vi "Measurement UI.vi"() -> ()   [LabVIEW 2021, in "audio_adc_frequencyResponseMeasurementUI.lvlib"]
uses:
  audio_adc_frequencyResponseMeasurementUI.lvlib
panel:
  in  "MeasGraphs":T1(tab)
  out "FrequencyResponseGraph":cluster{"X":dbl[], "Y":dbl[]}(graph) caption="AC"
  out "RMSLevelGraph":cluster{"X":dbl[], "Y":dbl[]}(graph) caption="AC"
  out "THDResponseGraph":cluster{"X":dbl[], "Y":dbl[]}(graph) caption="AC"
  out "THD+NResponseGraph":cluster{"X":dbl[], "Y":dbl[]}(graph) caption="AC"
  out "TimeDomainGraph":cluster{dbl, "dt":dbl, "Time domain":dbl[]}[](graph) caption="AC"
  in  "Bit clock edge sync":u32=1
  in  "Frame sync pulse width":u32=32
  in  "Frame length":u32=64
  in  "Data justification":u32 caption="Data Justification"
  in  "Endianness":u32
  in  "Channel 0 offset":u32=1
  in  "Bit depth":u32=24
  in  "Channel length":u32=32
  in  "Channel count per frame":u32=2
  in  "Frame sync edge for channel 0":u32=1
  out "Time domain plot sizes":i32[](array[numeric])
  out "THD+N response":dbl[](array[numeric])
  out "Frequency response":dbl[](array[numeric])
  out "Time domain":dbl[](array[numeric])
  out "dt":dbl
  out "RMS levels":dbl[](array[numeric])
  out "THD response":dbl[](array[numeric])
  out "Frequency steps":dbl[](array[numeric])
  in  "Configure Protocol Settings":bool
  in  "Analog source resource name":string(combo) caption="RESOURCE NAME"
  in  "Protocol capture resource name":string(combo) caption="RESOURCE NAME"
  in  "Data line":u16 caption="DATA LINE"
  in  "Channel":u32 caption="CHANNEL"
  in  "MeasSettingsOptions":i32(listbox)=-1
  in  "Settling time":dbl caption="SETTLING TIME" format="%#_6ps"
  in  "Settling cycles":i32 caption="SETTLING CYCLES"
  in  "Maximum harmonic":i32=5 caption="MAX HARMONIC"
  in  "DC Offset":dbl caption="DC OFFSET" format="%#_6pV"
  out "Protocol settings":string="Protocol settings"
  in  "Sample rate":dbl=44100.0 caption="SAMPLE RATE" format="%#.6pHz"
  in  "Frequency spacing":string(combo)="Logarithmic" caption="FREQUENCY SPACING"
  in  "Measurement duration":dbl=0.001 caption="MEASUREMENT DURATION" format="%#_6ps"
  in  "Measurement cycles":i32=10 caption="MEASUREMENT CYCLES"
  in  "Frequency steps":i32=20 caption="FREQUENCY STEPS"
  out "Analog source":string="Analog source "
  in  "Amplitude":dbl=-1.0 caption="AMPLITUDE" format="%#_6pdB"
  in  "Full scale range":dbl=2.825 caption="FULL SCALE RANGE" format="%.3pV"
  in  "Frequency stop":dbl=10000.0 caption="FREQUENCY STOP" format="%#_6pHz"
  in  "Frequency start":dbl=100.0 caption="FREQUENCY START" format="%#_6pHz"
  out "Measurement settings":string="Measurement settings"
  in  "MeasSettings":bool
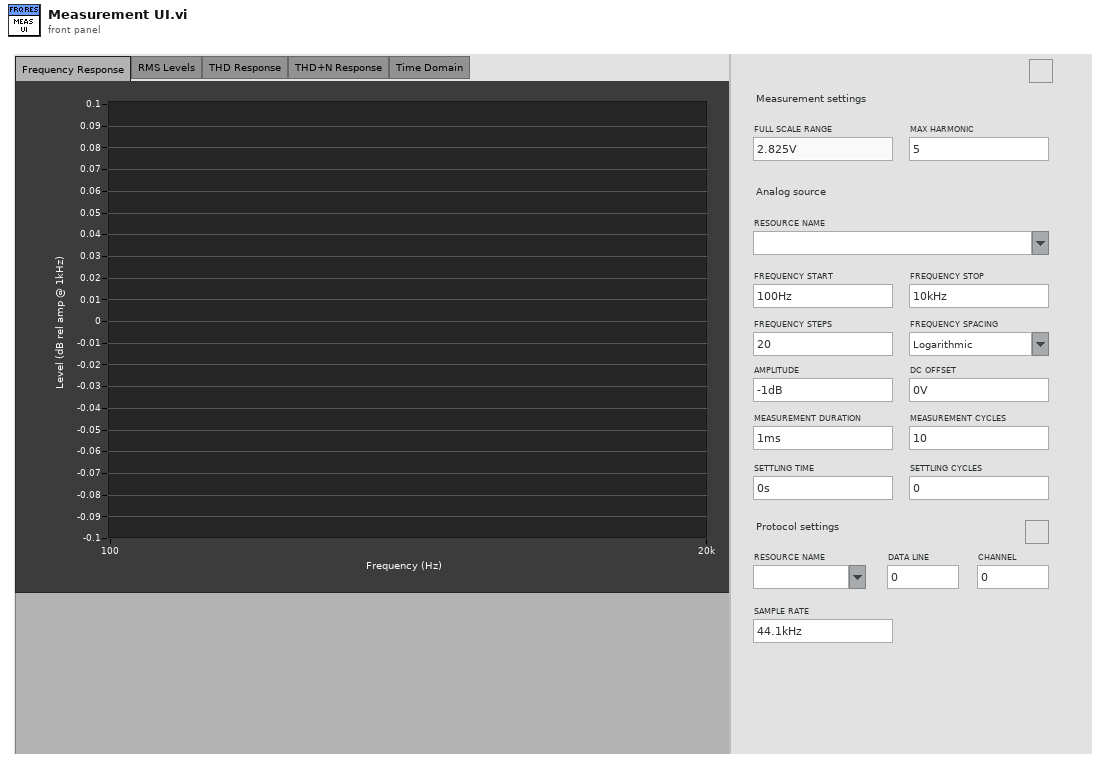
[diagram p1: front panel]
types:
  T1 = enum32{"Frequency Response", "RMS Levels", "THD Response", "THD+N Response", "Time Domain", "Hidden Controls"}
  T2 = enum16{"open", "replace", "create", "open or create", "replace or create", "replace or create with confirmation"}
  T3 = typedef "PDM Shared.lvlib/PCM Frame Sync Control.ctl" = cluster{"Frame Length":u16, "Frame Sync Pulse Width":u16, "Bit Clock Edge  Sync":T4}
  T4 = typedef "PDM Shared.lvlib/Digital Edge.ctl" = enum8{"Rising", "Falling"}
  T5 = typedef "PDM Shared.lvlib/PCM Data Format Configuration.ctl" = cluster{"Frame Sync Edge for Channel 0":T4, "Channel Count Per Frame":u8, "Channel Length":u16, "Bit Depth":u8, "Channel 0 Offset":u16, "Endianness":T6, "Data Justification":T7}
  T6 = typedef "PDM Shared.lvlib/PCM Bit Endianness.ctl" = enum16{"MSB First", "LSB First"}
  T7 = typedef "PDM Shared.lvlib/PCM Data Justification.ctl" = enum16{"Left Justified", "Right Justified"}
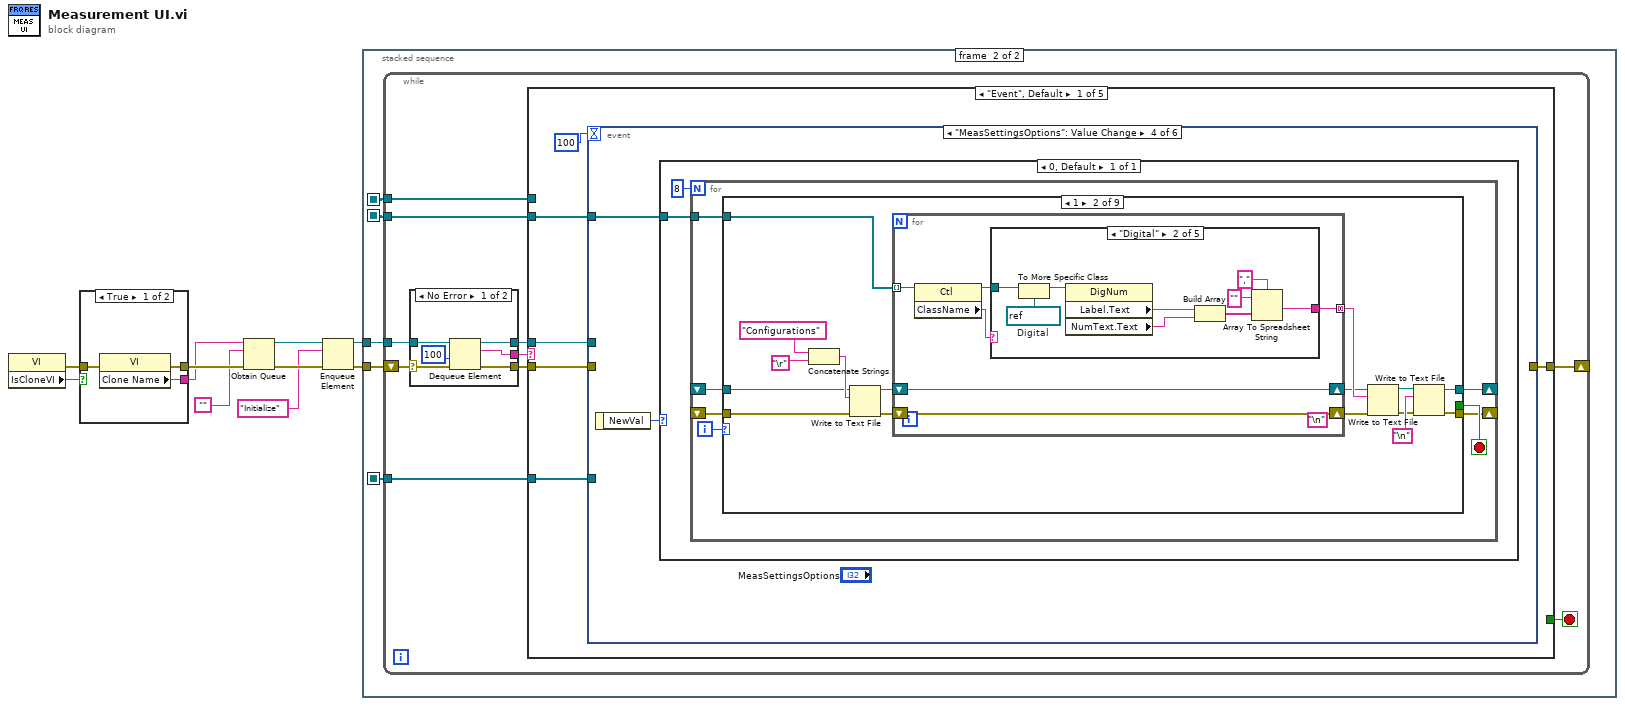
[diagram p0: block diagram]
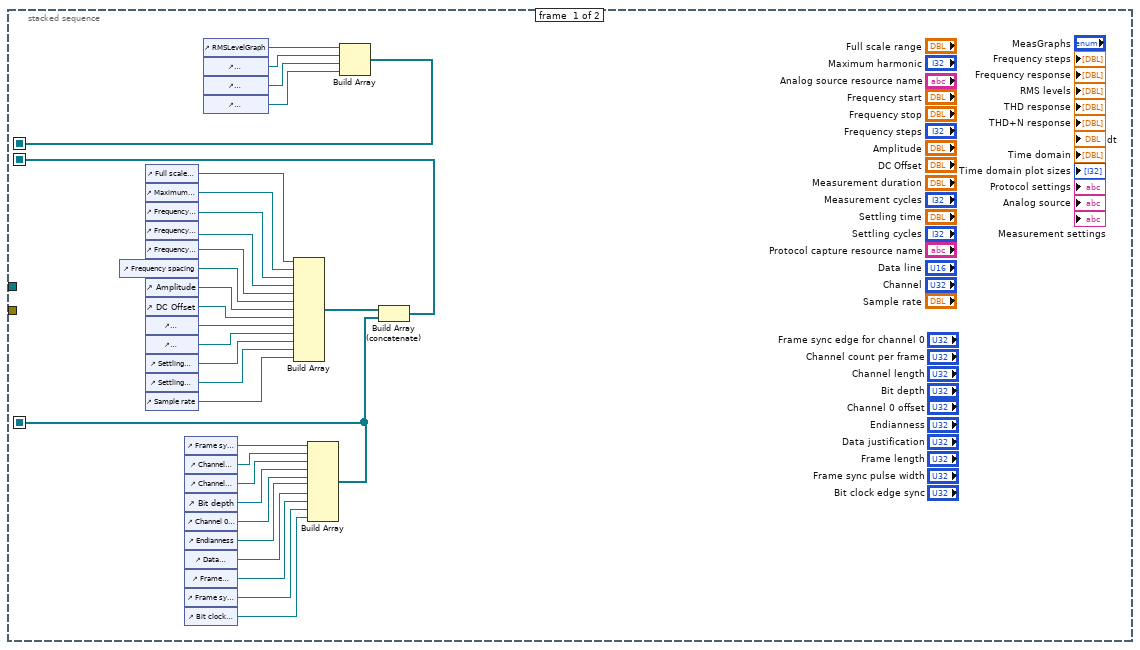
[diagram p2: hidden frame]
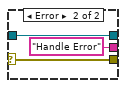
[diagram p3: hidden frame]
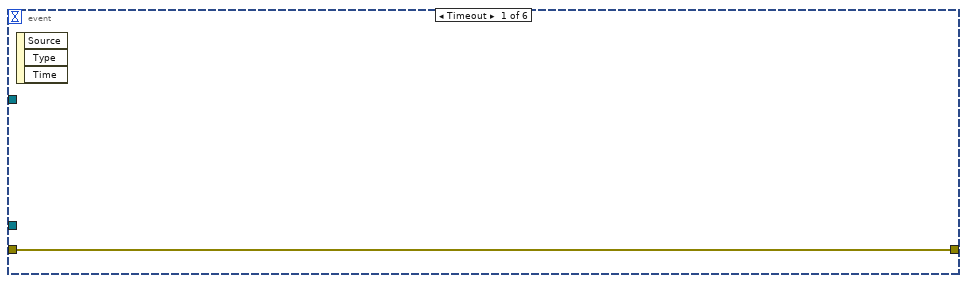
[diagram p4: hidden frame]
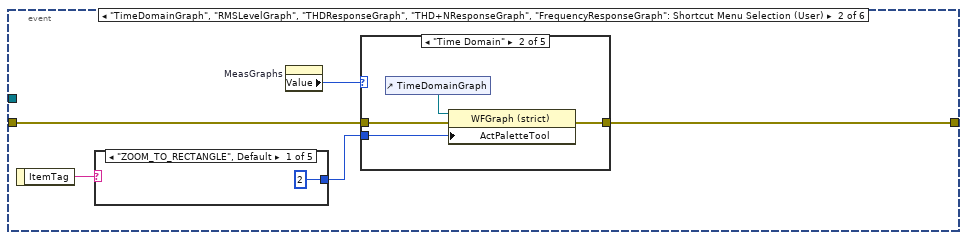
[diagram p5: hidden frame]
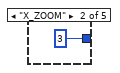
[diagram p6: hidden frame]
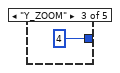
[diagram p7: hidden frame]
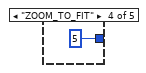
[diagram p8: hidden frame]
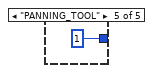
[diagram p9: hidden frame]
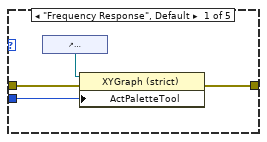
[diagram p10: hidden frame]
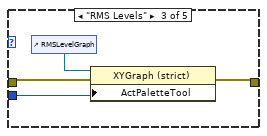
[diagram p11: hidden frame]
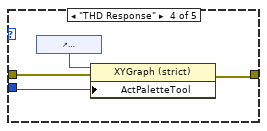
[diagram p12: hidden frame]
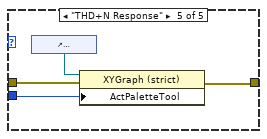
[diagram p13: hidden frame]
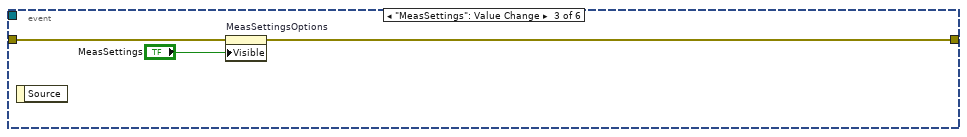
[diagram p14: hidden frame]
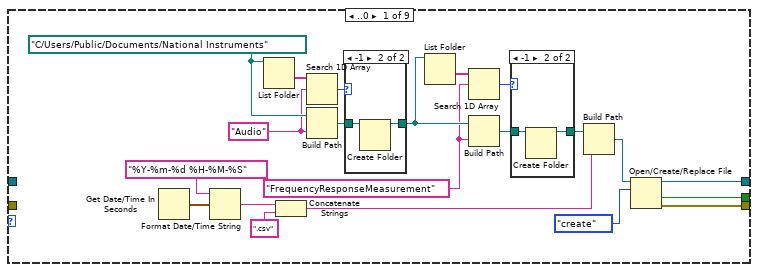
[diagram p15: hidden frame]
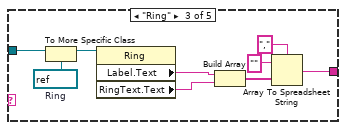
[diagram p19: hidden frame]
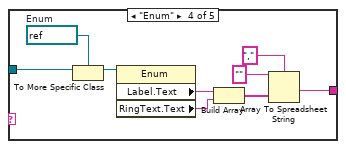
[diagram p20: hidden frame]
diagram:
  n1 = property class="VI"() -> (error out=w1:errorcluster, "IsCloneVI"=w2:bool)  [unwired: 2 in, 1 out]
  n2 = case shown="True" w2 {
    tunnel: [w13 w16] -> w10
    tunnel: [w12 w15] -> w9
    tunnel: w1 -> [w11 w14]
    frame True {
      n3 = property class="VI"(error in=w11) -> (error out=w13:errorcluster, "Clone Name"=w12:string)  [unwired: 1 in, 1 out]
    }
    frame False {
      n4 = property class="VI"(error in=w14) -> (error out=w16:errorcluster, "Name"=w15:string)  [unwired: 1 in, 1 out]
    }
  }
  n5 = Obtain Queue(name (unnamed)=w9, element data type="", error in (no error)=w10) -> (queue out=w6:refnum<queue>, error out=w8:errorcluster)  [unwired: 2 in, 1 out]
  n6 = Enqueue Element(queue=w6, element="Initialize", error in (no error)=w8) -> (queue out=w5:refnum<queue>, error out=w7:errorcluster)  [unwired: 1 in, 1 out]
  n7 = stacked-sequence {
    seq-local: [w18 _] -> [_ w48]
    seq-local: [w30 _] -> [_ w50]
    seq-local: [w17 _] -> [_ w49]
    tunnel: w7 -> [_ w52]
    tunnel: w5 -> [_ w51]
    frame #0 {
      n8 = control-ref of="Frequency spacing"() -> (w42:refnum<vi>)
      n9 = control-ref of="Full scale range"() -> (w47:refnum<vi>)
      n10 = control-ref of="Maximum harmonic"() -> (w46:refnum<vi>)
      n11 = control-ref of="Frequency start"() -> (w45:refnum<vi>)
      n12 = control-ref of="Frequency stop"() -> (w44:refnum<vi>)
      n13 = control-ref of="Frequency steps"() -> (w43:refnum<vi>)
      n14 = control-ref of="Amplitude"() -> (w36:refnum<vi>)
      n15 = control-ref of="DC Offset"() -> (w35:refnum<vi>)
      n16 = control-ref of="Measurement duration"() -> (w41:refnum<vi>)
      n17 = control-ref of="Measurement cycles"() -> (w40:refnum<vi>)
      n18 = control-ref of="Settling time"() -> (w39:refnum<vi>)
      n19 = control-ref of="Settling cycles"() -> (w38:refnum<vi>)
      n20 = control-ref of="Sample rate"() -> (w37:refnum<vi>)
      n21 = control-ref of="Frame sync edge for channel 0"() -> (w29:refnum<vi>)
      n22 = control-ref of="Channel count per frame"() -> (w28:refnum<vi>)
      n23 = control-ref of="Channel length"() -> (w27:refnum<vi>)
      n24 = control-ref of="Bit depth"() -> (w26:refnum<vi>)
      n25 = control-ref of="Channel 0 offset"() -> (w25:refnum<vi>)
      n26 = control-ref of="Endianness"() -> (w24:refnum<vi>)
      n27 = control-ref of="Data justification"() -> (w23:refnum<vi>)
      n28 = control-ref of="Frame length"() -> (w22:refnum<vi>)
      n29 = control-ref of="Frame sync pulse width"() -> (w21:refnum<vi>)
      n30 = control-ref of="Bit clock edge sync"() -> (w20:refnum<vi>)
      n31 = control-ref of="RMSLevelGraph"() -> (w34:refnum<vi>)
      n32 = control-ref of="THDResponseGraph"() -> (w33:refnum<vi>)
      n33 = control-ref of="THD+NResponseGraph"() -> (w32:refnum<vi>)
      n34 = control-ref of="FrequencyResponseGraph"() -> (w31:refnum<vi>)
      n35 = Build Array(w47, w46, w45, w44, w43, w42, w36, w35, w41, w40, w39, w38, w37) -> (w19:refnum<vi>[])
      n36 = Build Array(w29, w28, w27, w26, w25, w24, w23, w22, w21, w20) -> (w17:refnum<vi>[])
      n37 = Build Array(w34, w33, w32, w31) -> (w30:refnum<vi>[])
      n38 = Build Array (concatenate)(w19, w17) -> (w18:refnum<vi>[])
    }
    frame #1 {
      n39 = while {
        shift-right: [w57] -> _
        shift-left: w52 -> [w62]
        tunnel: w51 -> [w60]
        tunnel: w50 -> [w55]
        tunnel: w49 -> [w54]
        tunnel: w48 -> [w53]
        stop <- w56 stop-if-true
        n40 = case shown="No Error" w62 {
          selector: w62 -> [w68 w71]
          tunnel: [w67 w71] -> w61
          tunnel: w60 -> [w66 w70]
          tunnel: [w65 w70] -> w59
          tunnel: [w64 "Handle Error"] -> w58
          frame No Error {
            n41 = Dequeue Element(queue=w66, timeout in ms (-1)=100, error in (no error)=w68) -> (queue out=w65:refnum<queue>, element=w64:string, error out=w67:errorcluster)  [unwired: 1 out]
          }
          frame Error {
          }
        }
        n42 = case shown="\"Event\", Default" w58 {
          tunnel: w61 -> [w76 w394 w431 w458 w459]
          tunnel: w59 -> [w74 _ _ w456 _]
          tunnel: [w77 w394 w431 w453 w459] -> w57
          tunnel: [_ _ _ TRUE _] -> w56
          tunnel: w55 -> [_ _ w405 _ _]
          tunnel: w54 -> [w73 _ _ _ _]
          tunnel: w53 -> [w72 _ _ _ _]
          frame "Event", Default {
            n43 = event shown="[3] \"MeasSettingsOptions\": Value Change" {
              selector: _ -> [_ _ _ _ _ _]
              dyn-events: _ -> [_ _ _ _ _ _]
              timeout: 100 -> [_ _ _ _ _ _]
              tunnel: [w78 w79 w109 _ w381 w384] -> w77
              tunnel: w76 -> [w78 w81 w111 _ w381 w385]
              tunnel: w74 -> [_ _ _ _ _ w383]
              tunnel: w73 -> [_ _ _ _ w378 _]
              tunnel: w72 -> [_ _ _ w112 _ _]
              event Timeout {
                n44 = event-data() -> ()  [unwired: 1 in, 3 out]
              }
              event "TimeDomainGraph", "RMSLevelGraph", "THDResponseGraph", "THD+NResponseGraph", "FrequencyResponseGraph": Shortcut Menu Selection (User) {
                n45 = event-data() -> ("ItemTag"=w82:string)  [unwired: 1 in]
                n46 = case shown="\"ZOOM_TO_RECTANGLE\", Default" w82 {
                  tunnel: [2 3 4 5 1] -> w80
                  frame "ZOOM_TO_RECTANGLE", Default {
                  }
                  frame "X_ZOOM" {
                  }
                  frame "Y_ZOOM" {
                  }
                  frame "ZOOM_TO_FIT" {
                  }
                  frame "PANNING_TOOL" {
                  }
                }
                n47 = property on="MeasGraphs" class="TabCtl (strict)"() -> ("Value"=w83:T1)  [unwired: 2 in, 2 out]
                n48 = case shown="\"Time Domain\"" w83 {
                  tunnel: w81 -> [w92 w95 w99 w104 w108]
                  tunnel: w80 -> [w89 w94 w98 w101 w107]
                  tunnel: [w91 w93 w97 w103 w106] -> w79
                  frame "Frequency Response", Default {
                    n49 = control-ref of="FrequencyResponseGraph"() -> (w90:refnum<vi>)
                    n50 = property class="XYGraph (strict)"(reference=w90, error in=w92, "ActPaletteTool"=w89) -> (error out=w91:errorcluster)  [unwired: 1 out]
                  }
                  frame "Time Domain" {
                    n51 = control-ref of="TimeDomainGraph"() -> (w96:refnum<vi>)
                    n52 = property class="WFGraph (strict)"(reference=w96, error in=w95, "ActPaletteTool"=w94) -> (error out=w93:errorcluster)  [unwired: 1 out]
                  }
                  frame "RMS Levels" {
                    n53 = control-ref of="RMSLevelGraph"() -> (w100:refnum<vi>)
                    n54 = property class="XYGraph (strict)"(reference=w100, error in=w99, "ActPaletteTool"=w98) -> (error out=w97:errorcluster)  [unwired: 1 out]
                  }
                  frame "THD Response" {
                    n55 = control-ref of="THDResponseGraph"() -> (w102:refnum<vi>)
                    n56 = property class="XYGraph (strict)"(reference=w102, error in=w104, "ActPaletteTool"=w101) -> (error out=w103:errorcluster)  [unwired: 1 out]
                  }
                  frame "THD+N Response" {
                    n57 = control-ref of="THD+NResponseGraph"() -> (w105:refnum<vi>)
                    n58 = property class="XYGraph (strict)"(reference=w105, error in=w108, "ActPaletteTool"=w107) -> (error out=w106:errorcluster)  [unwired: 1 out]
                  }
                }
              }
              event "MeasSettings": Value Change {
                n59 = event-data() -> ()  [unwired: 1 in, 1 out]
                n60 = property on="MeasSettingsOptions" class="LstBox (strict)"(error in=w111, "Visible"="MeasSettings") -> (error out=w109:errorcluster)  [unwired: 1 in, 1 out]
              }
              event "MeasSettingsOptions": Value Change {
                n61 = event-data() -> ("NewVal"=w113:i32)  [unwired: 1 in]
                n62 = case shown="0, Default" w113 {
                  tunnel: w112 -> [w114]
                  frame 0, Default {
                    n63 = for {
                      N: 8 -> [_]
                      shift-right: [w120] -> _
                      shift-left: _ -> [w119]
                      shift-right: [w118] -> _
                      shift-left: _ -> [w117]
                      tunnel: w114 -> [w116]
                      i -> [w122]
                      stop <- w121 stop-if-true
                      n64 = case shown="1" w122 {
                        tunnel: [w136 _ _ _ _ _ _ _ _] -> w121
                        tunnel: [w142 w151 w215 w246 w278 w310 w340 refnum<file> refnum ("refnum out") w377] -> w120
                        tunnel: w119 -> [_ w162 w235 w267 w299 w331 w348 w375 w377]
                        tunnel: [w135 w152 w213 w244 w276 w308 w339 w373 w376] -> w118
                        tunnel: w117 -> [_ w160 w234 w266 w298 w330 w349 w372 w376]
                        tunnel: w116 -> [_ w150 _ _ _ _ _ _ _]
                        frame ..0 {
                          w131 = "FrequencyResponseMeasurement" ("prompt")
                          w138 = "Audio" ("prompt")
                          w141 = path "C:/Users/Public/Documents/National Instruments" ("base path")
                          n65 = Get Date/Time In Seconds() -> (seconds since 1Jan1904=w128:timestamp)
                          n66 = Format Date/Time String(time format string (%c)="%Y-%m-%d %H-%M-%S", seconds (now)=w128) -> (date/time string=w127:string)  [unwired: 1 in]
                          n67 = List Folder(path=w141) -> (folder names=w139:string[])  [unwired: 3 in, 3 out]
                          n68 = Concatenate Strings(w127, ".csv" ("string")) -> (w124:string)
                          n69 = Search 1D Array(1D array=w139, element=w138) -> (index of element=w137:i32)  [unwired: 1 in]
                          n70 = Build Path(base path=w141, name or relative path=w138) -> (appended path=w140:path)
                          n71 = case shown="-1" w137 {
                            tunnel: w140 -> [w147 w149]
                            tunnel: [w147 w148] -> w132
                            frame Default {
                            }
                            frame -1 {
                              n72 = Create Folder(path (use dialog)=w149) -> (created path=w148:path)  [unwired: 2 in, 2 out]
                            }
                          }
                          n73 = List Folder(path=w132) -> (folder names=w134:string[])  [unwired: 3 in, 3 out]
                          n74 = Search 1D Array(1D array=w134, element=w131) -> (index of element=w133:i32)  [unwired: 1 in]
                          n75 = Build Path(base path=w132, name or relative path=w131) -> (appended path=w130:path)
                          n76 = case shown="-1" w133 {
                            tunnel: w130 -> [w144 w146]
                            tunnel: [w144 w145] -> w125
                            frame Default {
                            }
                            frame -1 {
                              n77 = Create Folder(path (use dialog)=w146) -> (created path=w145:path)  [unwired: 2 in, 2 out]
                            }
                          }
                          n78 = Build Path(base path=w125, name or relative path=w124) -> (appended path=w123:path)
                          n79 = Open/Create/Replace File(file path (use dialog)=w123, operation (0:open)=T2."create") -> (refnum out=w142:refnum<file>, cancelled=w136:bool, error out=w135:errorcluster)  [unwired: 4 in]
                        }
                        frame 1 {
                          (unwired) "\n"
                          n80 = Concatenate Strings("Configurations" ("format string"), "\r") -> (w163:string)
                          n81 = Write to Text File(file (use dialog)=w162, text=w163, error in=w160) -> (refnum out=w159:refnum<file>, error out=w161:errorcluster)  [unwired: 1 in, 1 out]
                          n82 = for {
                            shift-right: [w171] -> w157
                            shift-left: w159 -> [w171]
                            shift-right: [w170] -> w156
                            shift-left: w161 -> [w170]
                            tunnel: [w169] -> w158 mode=concatenating
                            tunnel: w150 -> [w166] mode=indexing
                            n83 = property class="Ctl"(reference=w166) -> (reference out=w168:refnum<vi>, "ClassName"=w167:string)  [unwired: 1 in, 1 out]
                            n84 = case shown="\"Digital\"" w167 {
                              tunnel: [_ w175 w185 w194 w203] -> w169
                              tunnel: w168 -> [_ w173 w183 w198 w207]
                              frame Default {
                              }
                              frame "Digital" {
                                w172 = refnum<vi> refnum  # Digital
                                n85 = To More Specific Class(target class=w172, reference=w173) -> (specific class reference=w174:refnum<vi>)  [unwired: 1 in, 1 out]
                                n86 = property class="DigNum"(reference=w174) -> ("Label.Text"=w180:string, "NumText.Text"=w179:string)  [unwired: 1 in, 2 out]
                                n87 = Build Array(w180, w179) -> (w176:string[])
                                n88 = Array To Spreadsheet String(delimiter (Tab)=",", array=w176, 3:"" ("format string")) -> (spreadsheet string=w175:string)
                              }
                              frame "Ring" {
                                w182 = refnum<vi> refnum  # Ring
                                n89 = To More Specific Class(target class=w182, reference=w183) -> (specific class reference=w184:refnum<vi>)  [unwired: 1 in, 1 out]
                                n90 = property class="Ring"(reference=w184) -> ("Label.Text"=w181:string, "RingText.Text"=w189:string)  [unwired: 1 in, 2 out]
                                n91 = Build Array(w181, w189) -> (w186:string[])
                                n92 = Array To Spreadsheet String(delimiter (Tab)=",", array=w186, 3:"" ("format string")) -> (spreadsheet string=w185:string)
                              }
                              frame "Enum" {
                                w197 = refnum<vi> refnum  # Enum
                                n93 = To More Specific Class(target class=w197, reference=w198) -> (specific class reference=w193:refnum<vi>)  [unwired: 1 in, 1 out]
                                n94 = property class="Enum"(reference=w193) -> ("Label.Text"=w192:string, "RingText.Text"=w191:string)  [unwired: 1 in, 2 out]
                                n95 = Build Array(w192, w191) -> (w190:string[])
                                n96 = Array To Spreadsheet String(delimiter (Tab)=",", array=w190, 3:"" ("format string")) -> (spreadsheet string=w194:string)
                              }
                              frame "ComboBox" {
                                w206 = refnum<vi> refnum  # ComboBox
                                n97 = To More Specific Class(target class=w206, reference=w207) -> (specific class reference=w202:refnum<vi>)  [unwired: 1 in, 1 out]
                                n98 = property class="CmbBox"(reference=w202) -> ("Label.Text"=w201:string, "Value"=w200:string)  [unwired: 1 in, 2 out]
                                n99 = Build Array(w201, w200) -> (w199:string[])
                                n100 = Array To Spreadsheet String(delimiter (Tab)=",", array=w199, 3:"" ("format string")) -> (spreadsheet string=w203:string)
                              }
                            }
                          }
                          n101 = Write to Text File(file (use dialog)=w157, text=w158, error in=w156) -> (refnum out=w154:refnum<file>, error out=w153:errorcluster)  [unwired: 1 in, 1 out]
                          n102 = Write to Text File(file (use dialog)=w154, text="\n", error in=w153) -> (refnum out=w151:refnum<file>, error out=w152:errorcluster)  [unwired: 1 in, 1 out]
                        }
                        frame 2 {
                          w208 = "\r"
                          n103 = property on="FrequencyResponseGraph" class="XYGraph (strict)"() -> ("Value"=w210:cluster{"X":dbl[], "Y":dbl[]})  [unwired: 2 in, 2 out]
                          n104 = Concatenate Strings("Results" ("string"), w208, "Frequency Response" ("string"), w208) -> (w232:string)
                          n105 = Write to Text File(file (use dialog)=w235, text=w232, error in=w234) -> (refnum out=w228:refnum<file>, error out=w227:errorcluster)  [unwired: 1 in, 1 out]
                          n106 = Build Array("Frequency (Hz)", "Level (dB rel amp @ 1kHz)") -> (w231:string[])
                          n107 = Unbundle By Name(w210) -> ("X"=w219:dbl[], "Y"=w220:dbl[])
                          n108 = Array To Spreadsheet String(delimiter (Tab)=",", array=w231, 3:"" ("format string")) -> (spreadsheet string=w226:string)
                          n109 = for {
                            tunnel: w219 -> [w240] mode=indexing
                            tunnel: w220 -> [w236] mode=indexing
                            tunnel: [w237] -> w221 mode=indexing
                            n110 = Format Into String(w240) -> (resulting string=w238:string)  [unwired: 3 in, 1 out]
                            n111 = Format Into String(w236) -> (resulting string=w239:string)  [unwired: 3 in, 1 out]
                            n112 = Build Array(w238, w239) -> (w237:string[])
                          }
                          n113 = Write to Text File(file (use dialog)=w228, text=w226, error in=w227) -> (refnum out=w225:refnum<file>, error out=w224:errorcluster)  [unwired: 1 in, 1 out]
                          n114 = Array To Spreadsheet String(delimiter (Tab)=",", array=w221, 3:"" ("format string")) -> (spreadsheet string=w218:string)
                          n115 = Write to Text File(file (use dialog)=w225, text=w218, error in=w224) -> (refnum out=w217:refnum<file>, error out=w216:errorcluster)  [unwired: 1 in, 1 out]
                          n116 = Write to Text File(file (use dialog)=w217, text="\n", error in=w216) -> (refnum out=w215:refnum<file>, error out=w213:errorcluster)  [unwired: 1 in, 1 out]
                        }
                        frame 3 {
                          n117 = property on="RMSLevelGraph" class="XYGraph (strict)"() -> ("Value"=w241:cluster{"X":dbl[], "Y":dbl[]})  [unwired: 2 in, 2 out]
                          n118 = Concatenate Strings("RMS Level" ("string"), "\r") -> (w264:string)
                          n119 = Build Array("Frequency (Hz)", "Level (Vrms)") -> (w263:string[])
                          n120 = Write to Text File(file (use dialog)=w267, text=w264, error in=w266) -> (refnum out=w260:refnum<file>, error out=w259:errorcluster)  [unwired: 1 in, 1 out]
                          n121 = Array To Spreadsheet String(delimiter (Tab)=",", array=w263, 3:"" ("format string")) -> (spreadsheet string=w258:string)
                          n122 = Unbundle By Name(w241) -> ("X"=w251:dbl[], "Y"=w252:dbl[])
                          n123 = Write to Text File(file (use dialog)=w260, text=w258, error in=w259) -> (refnum out=w257:refnum<file>, error out=w256:errorcluster)  [unwired: 1 in, 1 out]
                          n124 = for {
                            tunnel: w251 -> [w272] mode=indexing
                            tunnel: w252 -> [w268] mode=indexing
                            tunnel: [w269] -> w253 mode=indexing
                            n125 = Format Into String(w272) -> (resulting string=w270:string)  [unwired: 3 in, 1 out]
                            n126 = Format Into String(w268) -> (resulting string=w271:string)  [unwired: 3 in, 1 out]
                            n127 = Build Array(w270, w271) -> (w269:string[])
                          }
                          n128 = Array To Spreadsheet String(delimiter (Tab)=",", array=w253, 3:"" ("format string")) -> (spreadsheet string=w250:string)
                          n129 = Write to Text File(file (use dialog)=w257, text=w250, error in=w256) -> (refnum out=w248:refnum<file>, error out=w247:errorcluster)  [unwired: 1 in, 1 out]
                          n130 = Write to Text File(file (use dialog)=w248, text="\n", error in=w247) -> (refnum out=w246:refnum<file>, error out=w244:errorcluster)  [unwired: 1 in, 1 out]
                        }
                        frame 4 {
                          n131 = Concatenate Strings("THD Response" ("string"), "\r") -> (w296:string)
                          n132 = property on="THDResponseGraph" class="XYGraph (strict)"() -> ("Value"=w273:cluster{"X":dbl[], "Y":dbl[]})  [unwired: 2 in, 2 out]
                          n133 = Build Array("Frequency (Hz)", "THD (dB)") -> (w295:string[])
                          n134 = Write to Text File(file (use dialog)=w299, text=w296, error in=w298) -> (refnum out=w292:refnum<file>, error out=w291:errorcluster)  [unwired: 1 in, 1 out]
                          n135 = Array To Spreadsheet String(delimiter (Tab)=",", array=w295, 3:"" ("format string")) -> (spreadsheet string=w290:string)
                          n136 = Unbundle By Name(w273) -> ("X"=w283:dbl[], "Y"=w284:dbl[])
                          n137 = Write to Text File(file (use dialog)=w292, text=w290, error in=w291) -> (refnum out=w289:refnum<file>, error out=w288:errorcluster)  [unwired: 1 in, 1 out]
                          n138 = for {
                            tunnel: w283 -> [w304] mode=indexing
                            tunnel: w284 -> [w300] mode=indexing
                            tunnel: [w301] -> w285 mode=indexing
                            n139 = Format Into String(w304) -> (resulting string=w302:string)  [unwired: 3 in, 1 out]
                            n140 = Format Into String(w300) -> (resulting string=w303:string)  [unwired: 3 in, 1 out]
                            n141 = Build Array(w302, w303) -> (w301:string[])
                          }
                          n142 = Array To Spreadsheet String(delimiter (Tab)=",", array=w285, 3:"" ("format string")) -> (spreadsheet string=w282:string)
                          n143 = Write to Text File(file (use dialog)=w289, text=w282, error in=w288) -> (refnum out=w280:refnum<file>, error out=w279:errorcluster)  [unwired: 1 in, 1 out]
                          n144 = Write to Text File(file (use dialog)=w280, text="\n", error in=w279) -> (refnum out=w278:refnum<file>, error out=w276:errorcluster)  [unwired: 1 in, 1 out]
                        }
                        frame 5 {
                          n145 = property on="THD+NResponseGraph" class="XYGraph (strict)"() -> ("Value"=w305:cluster{"X":dbl[], "Y":dbl[]})  [unwired: 2 in, 2 out]
                          n146 = Concatenate Strings("THD+N Response" ("string"), "\r") -> (w328:string)
                          n147 = Build Array("Frequency (Hz)", "THD+N (dB)") -> (w327:string[])
                          n148 = Write to Text File(file (use dialog)=w331, text=w328, error in=w330) -> (refnum out=w324:refnum<file>, error out=w323:errorcluster)  [unwired: 1 in, 1 out]
                          n149 = Array To Spreadsheet String(delimiter (Tab)=",", array=w327, 3:"" ("format string")) -> (spreadsheet string=w322:string)
                          n150 = Unbundle By Name(w305) -> ("X"=w315:dbl[], "Y"=w316:dbl[])
                          n151 = Write to Text File(file (use dialog)=w324, text=w322, error in=w323) -> (refnum out=w321:refnum<file>, error out=w320:errorcluster)  [unwired: 1 in, 1 out]
                          n152 = for {
                            tunnel: w315 -> [w336] mode=indexing
                            tunnel: w316 -> [w332] mode=indexing
                            tunnel: [w333] -> w317 mode=indexing
                            n153 = Format Into String(w336) -> (resulting string=w334:string)  [unwired: 3 in, 1 out]
                            n154 = Format Into String(w332) -> (resulting string=w335:string)  [unwired: 3 in, 1 out]
                            n155 = Build Array(w334, w335) -> (w333:string[])
                          }
                          n156 = Array To Spreadsheet String(delimiter (Tab)=",", array=w317, 3:"" ("format string")) -> (spreadsheet string=w314:string)
                          n157 = Write to Text File(file (use dialog)=w321, text=w314, error in=w320) -> (refnum out=w312:refnum<file>, error out=w311:errorcluster)  [unwired: 1 in, 1 out]
                          n158 = Write to Text File(file (use dialog)=w312, text="\n", error in=w311) -> (refnum out=w310:refnum<file>, error out=w308:errorcluster)  [unwired: 1 in, 1 out]
                        }
                        frame 6 {
                          n159 = Concatenate Strings("Time Domain" ("string"), "\r") -> (w361:string)
                          n160 = Write to Text File(file (use dialog)=w348, text=w361, error in=w349) -> (refnum out=w358:refnum<file>, error out=w357:errorcluster)  [unwired: 1 in, 1 out]
                          n161 = Build Array("Time (s)", "Amplitude (V)") -> (w360:string[])
                          n162 = property on="dt" class="DigNum (strict)"() -> ("Value"=w337:dbl)  [unwired: 2 in, 2 out]
                          n163 = property on="Time domain" class="Arr (strict)"() -> ("Value"=w338:dbl[])  [unwired: 2 in, 2 out]
                          n164 = Array To Spreadsheet String(delimiter (Tab)=",", array=w360, 3:"" ("format string")) -> (spreadsheet string=w356:string)
                          n165 = Write to Text File(file (use dialog)=w358, text=w356, error in=w357) -> (refnum out=w355:refnum<file>, error out=w354:errorcluster)  [unwired: 1 in, 1 out]
                          n166 = for {
                            tunnel: [w367] -> w351 mode=indexing
                            tunnel: w338 -> [w366] mode=indexing
                            tunnel: w337 -> [w364]
                            i -> [w365]
                            n167 = Multiply(x=w364, y=w365) -> (x*y=w363:dbl)
                            n168 = Format Into String(w363) -> (resulting string=w368:string)  [unwired: 3 in, 1 out]
                            n169 = Format Into String(w366) -> (resulting string=w369:string)  [unwired: 3 in, 1 out]
                            n170 = Build Array(w368, w369) -> (w367:string[])
                          }
                          n171 = Array To Spreadsheet String(delimiter (Tab)=",", array=w351, 3:"" ("format string")) -> (spreadsheet string=w350:string)
                          n172 = Write to Text File(file (use dialog)=w355, text=w350, error in=w354) -> (refnum out=w342:refnum<file>, error out=w341:errorcluster)  [unwired: 1 in, 1 out]
                          n173 = Write to Text File(file (use dialog)=w342, text="\n", error in=w341) -> (refnum out=w340:refnum<file>, error out=w339:errorcluster)  [unwired: 1 in, 1 out]
                        }
                        frame 7 {
                          w371 = FALSE ("Visible")
                          n174 = Close File(refnum=w375, error in=w372) -> (error out=w373:errorcluster)  [unwired: 1 out]
                          n175 = property on="MeasSettingsOptions" class="LstBox (strict)"("Visible"=w371, "Value"=-1 ("MeasSettingsOptions")) -> ()  [unwired: 2 in, 2 out]
                          n176 = property on="MeasSettings" class="Bool (strict)"("Value"=w371) -> ()  [unwired: 2 in, 2 out]
                        }
                        frame Default {
                        }
                      }
                    }
                  }
                }
              }
              event "Configure Protocol Settings": Value Change {
                n177 = event-data() -> ()  [unwired: 1 in, 1 out]
                n178 = call "Protocol Settings.vi"() -> ("Frame sync clock control"=w379:T3, "PDM data configuration"=w380:T5)  [unwired: 10 in]
                n179 = call "Update Protocol UI Controls.vi"("Frame Sync Clock Control"=w379, "PCM Data Configuration"=w380, "Control references"=w378) -> ()  [unwired: 9 in]
              }
              event Panel Close? {
                n180 = event-data() -> ()  [unwired: 1 in, 4 out]
                n181 = Enqueue Element(queue=w383, element="Exit", error in (no error)=w385) -> (error out=w384:errorcluster)  [unwired: 1 in, 2 out]
                n182 = event-data("Discard?"=TRUE) -> ()  [unwired: 1 in, 1 out]
              }
            }
          }
          frame "Initialize" {
            w387 = 2 ("Palette:Active Tool")
            n183 = control-ref of="TimeDomainGraph"() -> (w389:refnum<vi>)
            n184 = control-ref of="FrequencyResponseGraph"() -> (w390:refnum<vi>)
            n185 = control-ref of="THDResponseGraph"() -> (w392:refnum<vi>)
            n186 = control-ref of="RMSLevelGraph"() -> (w391:refnum<vi>)
            n187 = control-ref of="THD+NResponseGraph"() -> (w388:refnum<vi>)
            n188 = Build Array(w390, w392, w391, w388) -> (w393:refnum<vi>[])
            n189 = for {
              tunnel: w393 -> [w403] mode=indexing
              tunnel: w387 -> [w402]
              n190 = property class="XYGraph (strict)"(reference=w403, "ActPaletteTool"=w402) -> ()  [unwired: 1 in, 2 out]
            }
            n191 = stacked-sequence {
              frame #0 {
                n192 = call "Detected DSGs.vi"() -> ("AO channels"=w397:string[])  [unwired: 11 in]
                n193 = Index Array(array=w397, index=0) -> (element=w396:string)
                n194 = property on="Analog source resource name" class="CmbBox"("Strings[]"=w397, "Value"=w396) -> ()  [unwired: 2 in, 2 out]
              }
              frame #1 {
                n195 = call "Detected PDMs.vi"() -> ("PDM devices"=w400:string[])  [unwired: 11 in]
                n196 = Index Array(array=w400, index=0) -> (element=w399:string)
                n197 = property on="Protocol capture resource name" class="CmbBox"("Strings[]"=w400, "Value"=w399) -> ()  [unwired: 2 in, 2 out]
              }
              frame #2 {
                n198 = property on="Frequency steps" class="DigNum (strict)"("Val(Sgnl)"=20 ("Value (Signaling)")) -> ()  [unwired: 2 in, 2 out]
              }
            }
            n199 = property class="WFGraph (strict)"(reference=w389, "ActPaletteTool"=w387) -> ()  [unwired: 1 in, 2 out]
          }
          frame "Post UI Update" {
            w410 = u32[] [15787074, 5682409, 15535092, 40563, 13983232, 35009, 15113984, 13400487, 15993633, 10221451, 8148942, 15869817, 32914, 10196480, 6271923, 16355671]  # Plot colors
            # "This case will be triggered, after framework updates the User interface with result values."
            n200 = local read "Time domain plot sizes"() -> (w412:i32[])
            n201 = property on="TimeDomainGraph" class="WFGraph (strict)"() -> ("Value"=w416:cluster{dbl, "dt":dbl, "Time domain":dbl[]}[])  [unwired: 2 in, 2 out]
            n202 = Not Equal?(x="Linear", y="Frequency spacing") -> (x != y?=w407:bool)
            n203 = Boolean To (0,1)(Boolean=w407) -> (0, 1=w404:i16)
            n204 = Array Size(array=w416) -> (size(s)=w414:i32)
            n205 = for {
              tunnel: w405 -> [w433] mode=indexing
              tunnel: w404 -> [w432]
              n206 = property class="XYGraph (strict)"(reference=w433, "XScale.Mapping Mode"=w432) -> ()  [unwired: 1 in, 2 out]
            }
            n207 = Array Size(array=w412) -> (size(s)=w415:i32)
            n208 = Not Equal?(x=w414, y=w415) -> (x != y?=w413:bool)
            n209 = case shown="True" w413 {
              tunnel: w412 -> [w434 w435]
              tunnel: [w434 w435] -> w411
              tunnel: w410 -> [_ w436]
              frame False {
              }
              frame True {
                n210 = for {
                  tunnel: w435 -> [_] mode=indexing
                  tunnel: w436 -> [w439]
                  i -> [w441]
                  n211 = Quotient & Remainder(x=w441, y=16) -> (x-y*floor(x/y)=w438:i32)  [unwired: 1 out]
                  n212 = Index Array(array=w439, index=w438) -> (element=w437:u32)
                  n213 = property on="TimeDomainGraph" class="WFGraph (strict)"("Active Plot"=w441, "Plot.Plot Color"=w437) -> ()  [unwired: 2 in, 2 out]
                }
              }
            }
            n214 = local read "Frequency response"() -> (w430:dbl[])
            n215 = local read "THD+N response"() -> (w423:dbl[])
            n216 = local read "Frequency steps"() -> (w428:dbl[])
            n217 = local read "THD response"() -> (w424:dbl[])
            n218 = local read "RMS levels"() -> (w421:dbl[])
            n219 = Bundle By Name(cluster=cluster{"X":dbl[], "Y":dbl[]} {"X"=[], "Y"=[]} ("THD vs Amplitude"), "X"=w428) -> (w420:cluster{"X":dbl[], "Y":dbl[]})
            n220 = Bundle By Name(cluster=w420, "Y"=w421) -> (→"RMSLevelGraph":cluster{"X":dbl[], "Y":dbl[]})
            n221 = local read "Time domain"() -> (w419:dbl[])
            n222 = Bundle By Name(cluster=w420, "Y"=w424) -> (→"THDResponseGraph":cluster{"X":dbl[], "Y":dbl[]})
            n223 = Bundle By Name(cluster=w420, "Y"=w423) -> (→"THD+NResponseGraph":cluster{"X":dbl[], "Y":dbl[]})
            n224 = local read "dt"() -> (w418:dbl)
            n225 = Bundle By Name(cluster=w420, "Y"=w430) -> (→"FrequencyResponseGraph":cluster{"X":dbl[], "Y":dbl[]})
            n226 = for {
              tunnel: w411 -> [w449] mode=indexing
              shift-right: [w445] -> _
              shift-left: w419 -> [w451]
              tunnel: w418 -> [w446]
              shift-right: [w448] -> _
              shift-left: 0 -> [w450]
              tunnel: [w444] -> w406 mode=indexing
              n227 = Multiply(x=w446, y=w450) -> (x*y=w447:dbl)
              n228 = Add(x=w450, y=w449) -> (x+y=w448:i32)
              n229 = Delete From Array(array=w451, length=w449, index=0) -> (deleted portion=w442:dbl[], array with subset deleted=w445:dbl[])
              n230 = Bundle(w447, "dt"=w446, "Time domain"=w442) -> (w444:cluster{dbl, "dt":dbl, "Time domain":dbl[]})  [unwired: 1 in]
            }
            "TimeDomainGraph" <- w406
          }
          frame "Exit" {
            # "This case is triggered to close the User Interface from framework"
            n231 = Flush Queue(queue=w456, error in (no error)=w458) -> (queue out=w455:refnum<queue>, error out=w454:errorcluster)  [unwired: 1 out]
            n232 = Release Queue(queue=w455, force destroy? (F)=TRUE, error in (no error)=w454) -> (error out=w453:errorcluster)  [unwired: 2 out]
          }
          frame "Handle Error" {
          }
        }
      }
    }
  }
